vi "Window Comparisons.vi"() -> ()   [LabVIEW 2025]
uses:
  <vilib>/Analysis/2dsp.llb/Real FFT.vi
  <vilib>/Analysis/0measdsp.llb/Scaled Time Domain Window (DBL).vi
  <vilib>/Analysis/NI_AALBase.lvlib
  <vilib>/Analysis/NI_AALPro.lvlib
panel:
  in  "Kaiser Parameter":dbl=300.0 min=0.0001 max=300.0 step=0.1 format="%#_13g"
  in  "add noise":bool
  in  "100dB Zoom \nSpectrum Scale":bool
  in  "Window":u32(ring) items=["Rectangle"=0, "Hanning"=1, "Hamming"=2, "Blackman-Harris"=3, "Exact Blackman"=4, "Blackman"=5, "Flat Top"=6, "4 Term B-Harris "=7, "7 Term B-Harris"=8, "Low Sidelobe"=9, "Blackman Nuttall"=11, "Triangle"=30, "Bartlett-Hanning"=31, "Bohman"=32, "Parzen"=33, "Welch"=34, "Kaiser"=60, "Dolph-Chebyshev"=61, "Gaussian"=62]
  in  "Cylcles 2":dbl=13.0 min=0.0 max=200.0 format="%.1g"
  in  "Cylcles 1":dbl=13.0 min=0.0 max=200.0 step=1.0 format="%.1g"
  out "The Signal":dbl[](graph)
  out "The Spectrum":dbl[](graph)
  out "The Windowed Signal":dbl[][](graph)
  out "The Windowed Spectrum":dbl[](graph)
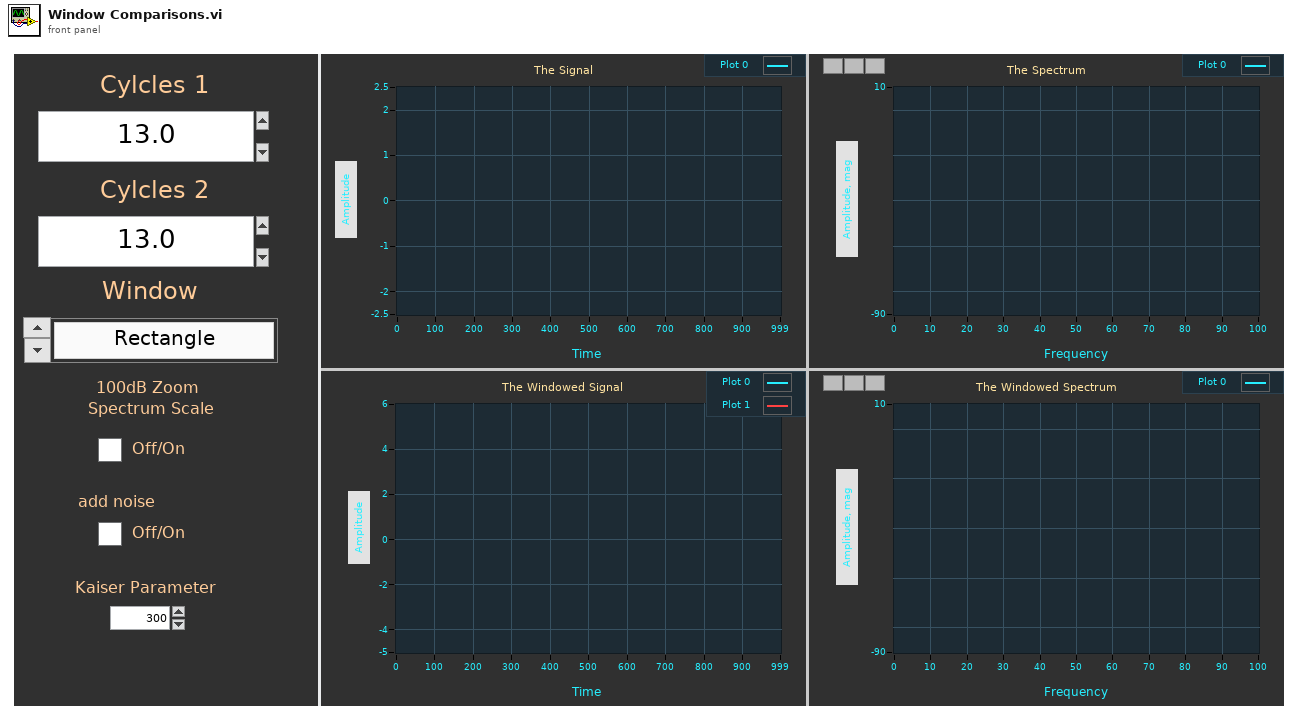
[diagram p1: front panel]
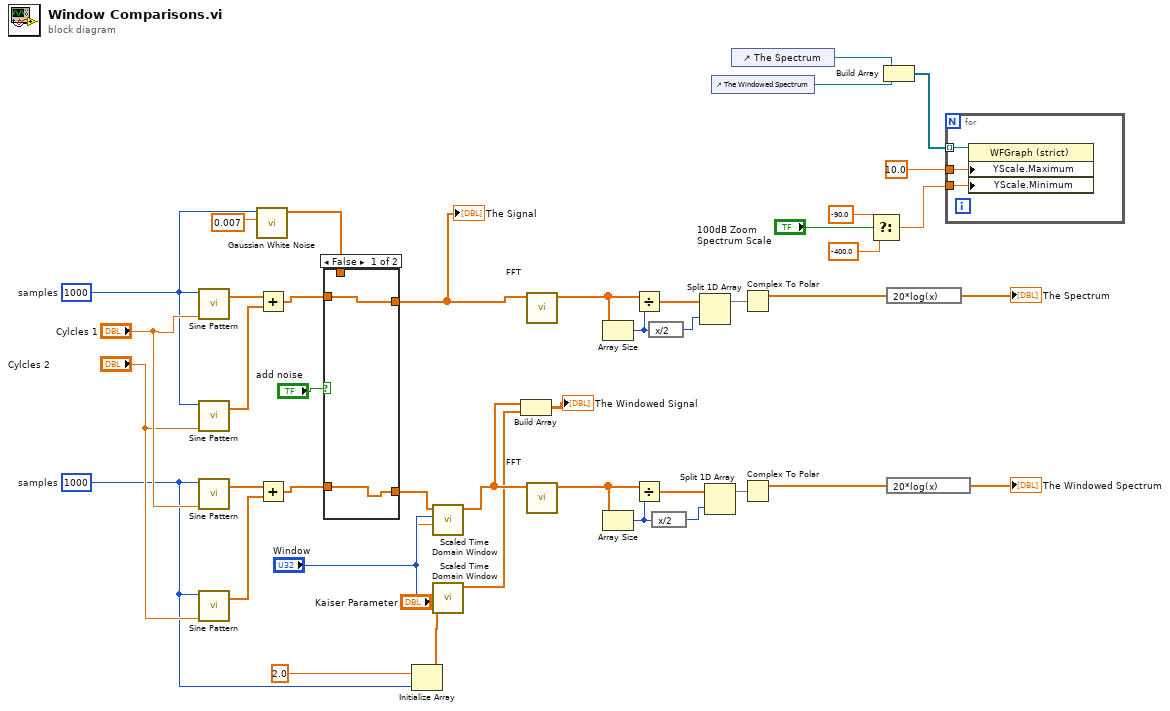
[diagram p0: block diagram]
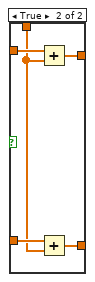
[diagram p2: hidden frame]
diagram:
  w13 = 1000  # samples
  w3 = 1000  # samples
  n1 = call <vilib>:"Sine Pattern.vi"("cycles"="Cylcles 1", "samples"=w3) -> ("Sinusoidal Pattern"=w42:dbl[])  [unwired: 2 in, 1 out]
  n2 = call <vilib>:"Sine Pattern.vi"("cycles"="Cylcles 2", "samples"=w3) -> ("Sinusoidal Pattern"=w40:dbl[])  [unwired: 2 in, 1 out]
  n3 = call <vilib>:"Sine Pattern.vi"("cycles"="Cylcles 1", "samples"=w13) -> ("Sinusoidal Pattern"=w38:dbl[])  [unwired: 2 in, 1 out]
  n4 = call <vilib>:"Sine Pattern.vi"("cycles"="Cylcles 2", "samples"=w13) -> ("Sinusoidal Pattern"=w39:dbl[])  [unwired: 2 in, 1 out]
  n5 = call <vilib>:"Gaussian White Noise.vi"("standard deviation"=0.007, "samples"=w3) -> ("Gaussian noise pattern"=w5:dbl[])  [unwired: 8 in, 1 out]
  n6 = Add(x=w42, y=w40) -> (x+y=w41:dbl[])
  n7 = Add(x=w38, y=w39) -> (x+y=w25:dbl[])
  n8 = case shown="False" "add noise" {
    tunnel: w41 -> [w46 w51]
    tunnel: w25 -> [w45 w50]
    tunnel: [w45 w49] -> w7
    tunnel: [w46 w48] -> w6
    tunnel: w5 -> [_ w47]
    frame False {
    }
    frame True {
      n9 = Add(x=w51, y=w47) -> (x+y=w48:dbl[])
      n10 = Add(x=w50, y=w47) -> (x+y=w49:dbl[])
    }
  }
  "The Signal" <- w6
  n11 = Initialize Array(2.0 ("element"), w13) -> (w11:dbl[])
  n12 = call-poly <vilib>:"Scaled Time Domain Window.vi"("window parameter"="Kaiser Parameter", "window"="Window", "X"=w7) -> ("Windowed X"=w24:dbl[])  [unwired: 6 in, 2 out]
  n13 = call-poly <vilib>:"Scaled Time Domain Window.vi"("window parameter"="Kaiser Parameter", "window"="Window", "X"=w11) -> ("Windowed X"=w9:dbl[])  [unwired: 6 in, 2 out]
  n14 = Build Array(w24, w9) -> (→"The Windowed Signal":dbl[][])
  n15 = call-poly <vilib>:"FFT.vi"("X"=w6) -> ("FFT {X}"=w44:cdb[])  [unwired: 9 in, 1 out]
  n16 = call-poly <vilib>:"FFT.vi"("X"=w24) -> ("FFT {X}"=w36:cdb[])  [unwired: 9 in, 1 out]
  n17 = Array Size(array=w44) -> (size(s)=w32:i32)
  n18 = Array Size(array=w36) -> (size(s)=w33:i32)
  n19 = Divide(x=w44, y=w32) -> (x/y=w43:cdb[])
  n20 = Divide(x=w36, y=w33) -> (x/y=w37:cdb[])
  n21 = expression code="x/2"(w32) -> (w30:i32)
  n22 = expression code="x/2"(w33) -> (w31:i32)
  n23 = Split 1D Array(array=w43, index=w30) -> (first subarray=w35:cdb[])  [unwired: 1 out]
  n24 = Split 1D Array(array=w37, index=w31) -> (first subarray=w34:cdb[])  [unwired: 1 out]
  n25 = control-ref of="The Windowed Spectrum"() -> (w15:refnum<vi>)
  n26 = control-ref of="The Spectrum"() -> (w16:refnum<vi>)
  n27 = Complex To Polar(r * e^(i*theta)=w35) -> (r=w29:dbl[])  [unwired: 1 out]
  n28 = Complex To Polar(r * e^(i*theta)=w34) -> (r=w28:dbl[])  [unwired: 1 out]
  n29 = Select(t=-90.0 ("Y Scale.Range:Maximum"), s="100dB Zoom \nSpectrum Scale", f=-400.0 ("Y Scale.Range:Maximum")) -> (s? t:f=w17:dbl)
  n30 = Build Array(w16, w15) -> (w14:refnum<vi>[])
  n31 = expression code="20*log(x)"(w29) -> (→"The Spectrum":dbl[])
  n32 = expression code="20*log(x)"(w28) -> (→"The Windowed Spectrum":dbl[])
  n33 = for {
    tunnel: 10.0 ("Y Scale.Range:Maximum") -> [w54]
    tunnel: w17 -> [w53]
    tunnel: w14 -> [w52] mode=indexing
    n34 = property on="Property Node" class="WFGraph (strict)"(reference=w52, "YScale.Maximum"=w54, "YScale.Minimum"=w53) -> ()  [unwired: 1 in, 2 out]
  }
